vi "Get Tag Value.vi"(3 "Tag Code":u16, 4 "DirEntries":T1[](array[typedef]), 5 "Image Data in":u8[](array[numeric])) -> (0 "Multiple Values":u64[](array[numeric]), 1 "Single Value":u32, 2 "Image Data out":u8[](array[numeric]))   [LabVIEW 2012, in "TIFF File Reader.lvlib"]
doc: "Reads a single specific tag in the array of tags returned by Read Image File Directory.vi and returns the associated data (either a single value or multiple values). The definition and meaning of the various tags is given in the tiff specifications."
uses:
  TIFF File Reader.lvlib
  IFD Entry.ctl
  FieldTypes.ctl
  Globals.vi
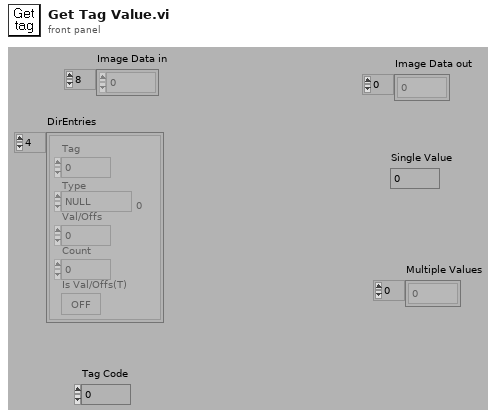
[diagram p1: front panel]
types:
  T1 = typedef "TIFF File Reader.lvlib/IFD Entry.ctl" = cluster{"Tag":u16, "Type":T2, "Count":u32, "Val/Offs":u32, "Is Val/Offs(T)":bool}
  T2 = typedef "TIFF File Reader.lvlib/FieldTypes.ctl" = enum16{"NULL", "U8", "ASCII7", "U16", "U32", "RATIONAL", "SByte(I8)", "Undef(8Bit)", "I16", "I32", "SRat(4B:4B)", "SGL(4Byte)", "DBL(8Byte)"}
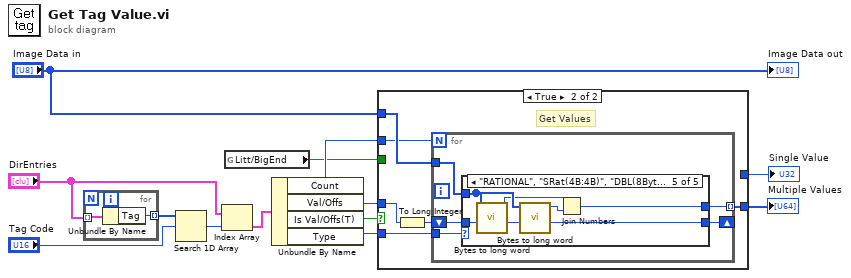
[diagram p0: block diagram]
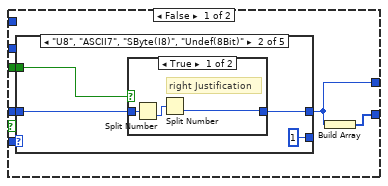
[diagram p2: hidden frame]
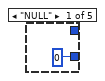
[diagram p3: hidden frame]
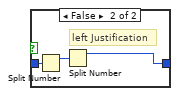
[diagram p4: hidden frame]
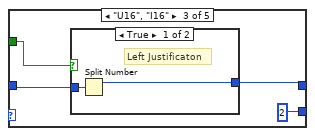
[diagram p5: hidden frame]
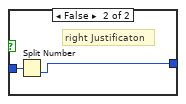
[diagram p6: hidden frame]
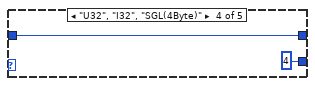
[diagram p7: hidden frame]
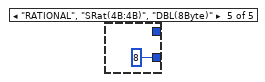
[diagram p8: hidden frame]
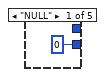
[diagram p9: hidden frame]
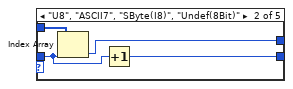
[diagram p10: hidden frame]
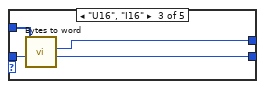
[diagram p11: hidden frame]
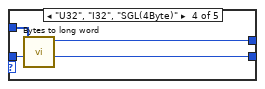
[diagram p12: hidden frame]
diagram:
  n1 = for {
    tunnel: "DirEntries" -> [w15] mode=indexing
    tunnel: [w14] -> w6 mode=indexing
    n2 = Unbundle By Name(w15) -> ("Tag"=w14:u16)
  }
  n3 = Search 1D Array(1D array=w6, element="Tag Code") -> (index of element=w4:i32)  [unwired: 1 out]
  n4 = Index Array(array="DirEntries", index=w4) -> (element=w12:T1)
  n5 = global read "Globals.vi" "Litt/BigEnd"() -> (w1:bool)
  n6 = Unbundle By Name(w12) -> ("Count"=w3:u32, "Val/Offs"=w10:u32, "Is Val/Offs(T)"=w11:bool, "Type"=w9:T2)
  n7 = case shown="True" w11 {
    tunnel: w10 -> [w18 w46]
    tunnel: w9 -> [w19 w47]
    tunnel: "Image Data in" -> [_ w45]
    tunnel: [w20 w48] -> w7
    tunnel: w3 -> [_ w44]
    tunnel: [w17 _] -> w2
    tunnel: w1 -> [w16 _]
    frame False {
      n8 = case shown="\"U8\", \"ASCII7\", \"SByte(I8)\", \"Undef(8Bit)\"" w19 {
        tunnel: [0 1 2 4 8] -> _
        tunnel: w18 -> [_ w24 w34 w40 _]
        tunnel: [_ w23 w33 w40 _] -> w17
        tunnel: w16 -> [_ w22 w32 _ _]
        frame "NULL" {
        }
        frame "U8", "ASCII7", "SByte(I8)", "Undef(8Bit)" {
          n9 = case shown="True" w22 {
            tunnel: w24 -> [w28 w31]
            tunnel: [w26 w29] -> w23
            frame True {
              # "right Justification"
              n10 = Split Number(x=w28) -> (lo(x)=w27:u16)  [unwired: 1 out]
              n11 = Split Number(x=w27) -> (lo(x)=w26:u8)  [unwired: 1 out]
            }
            frame False {
              # "left Justification"
              n12 = Split Number(x=w31) -> (hi(x)=w30:u16)  [unwired: 1 out]
              n13 = Split Number(x=w30) -> (hi(x)=w29:u8)  [unwired: 1 out]
            }
          }
        }
        frame "U16", "I16" {
          n14 = case shown="True" w32 {
            tunnel: w34 -> [w37 w39]
            tunnel: [w36 w38] -> w33
            frame True {
              # "Left Justificaton"
              n15 = Split Number(x=w37) -> (hi(x)=w36:u16)  [unwired: 1 out]
            }
            frame False {
              # "right Justificaton"
              n16 = Split Number(x=w39) -> (lo(x)=w38:u16)  [unwired: 1 out]
            }
          }
        }
        frame "U32", "I32", "SGL(4Byte)" {
        }
        frame "RATIONAL", "SRat(4B:4B)", "DBL(8Byte)" {
        }
      }
      n17 = Build Array(w17) -> (w20:u32[])
    }
    frame True {
      # "Get Values"
      n18 = To Long Integer(number=w46) -> (32bit integer=w43:i32)
      n19 = for {
        N: w44 -> [_]
        tunnel: w45 -> [w52]
        tunnel: w47 -> [w53]
        tunnel: [w51] -> w48 mode=indexing
        shift-right: [w49] -> _
        shift-left: w43 -> [w50]
        n20 = case shown="\"RATIONAL\", \"SRat(4B:4B)\", \"DBL(8Byte)\"" w53 {
          tunnel: w52 -> [_ w58 w60 w66 w71]
          tunnel: w50 -> [_ w56 w62 w65 w73]
          tunnel: [_ w57 w59 w64 w68] -> w51
          tunnel: [0 ("Index+2") w55 w61 w63 w67] -> w49
          frame "NULL" {
          }
          frame "U8", "ASCII7", "SByte(I8)", "Undef(8Bit)" {
            n21 = Index Array(array=w58, index=w56) -> (element=w57:u8)
            n22 = Increment(x=w56) -> (x+1=w55:i32)
          }
          frame "U16", "I16" {
            n23 = call "Bytes to word.vi"("Index"=w62, "Image Data in"=w60) -> ("Index+2"=w61:i32, "Word"=w59:u16)  [unwired: 2 in, 4 out]
          }
          frame "U32", "I32", "SGL(4Byte)" {
            n24 = call "Bytes to long word.vi"("Index"=w65, "Image Data in"=w66) -> ("Index+4"=w63:i32, "U32"=w64:u32)  [unwired: 6 out]
          }
          frame "RATIONAL", "SRat(4B:4B)", "DBL(8Byte)" {
            n25 = call "Bytes to long word.vi"("Index"=w73, "Image Data in"=w71) -> ("Index+4"=w72:i32, "U32"=w70:u32)  [unwired: 6 out]
            n26 = call "Bytes to long word.vi"("Index"=w72, "Image Data in"=w71) -> ("Index+4"=w67:i32, "U32"=w69:u32)  [unwired: 6 out]
            n27 = Join Numbers(hi=w70, lo=w69) -> ((hi.lo)=w68:u64)
          }
        }
      }
    }
  }
  "Multiple Values" <- w7
  "Single Value" <- w2
  "Image Data out" <- "Image Data in"
